vi "niDTS BT Rx Test INC Default Limits.vi"() -> ()   [LabVIEW 2015, in "niDTS BT.lvlib"]
uses:
  niDTS BT.lvlib
  niDTS BT Rx Test INC Results.ctl
panel:
  in  "Default BT RX LE USL":T1={"Total Packets Received (LE)"=2147483647, "Packets Sent (LE)"=inf, "Good Packets"=inf, "Packet Error Rate (%)"=30.8, "Error Bits"=4294967295, "Good Bits"=4294967295, "Total Received Bits"=4294967295, "Bit Error Rate (%)"=100.0}
  in  "Default BT RX LE LSL":T1
  in  "Default BT RX EDR USL":T1={"Total Packets Received (LE)"=2147483647, "Packets Sent (LE)"=inf, "Good Packets"=inf, "Packet Error Rate (%)"=100.0, "Error Bits"=4294967295, "Good Bits"=4294967295, "Total Received Bits"=4294967295, "Bit Error Rate (%)"=0.1}
  in  "Default BT RX EDR LSL":T1
  in  "Default BT RX BDR USL":T1={"Total Packets Received (LE)"=2147483647, "Packets Sent (LE)"=inf, "Good Packets"=inf, "Packet Error Rate (%)"=100.0, "Error Bits"=4294967295, "Good Bits"=4294967295, "Total Received Bits"=4294967295, "Bit Error Rate (%)"=0.007}
  in  "Default BT RX BDR LSL":T1
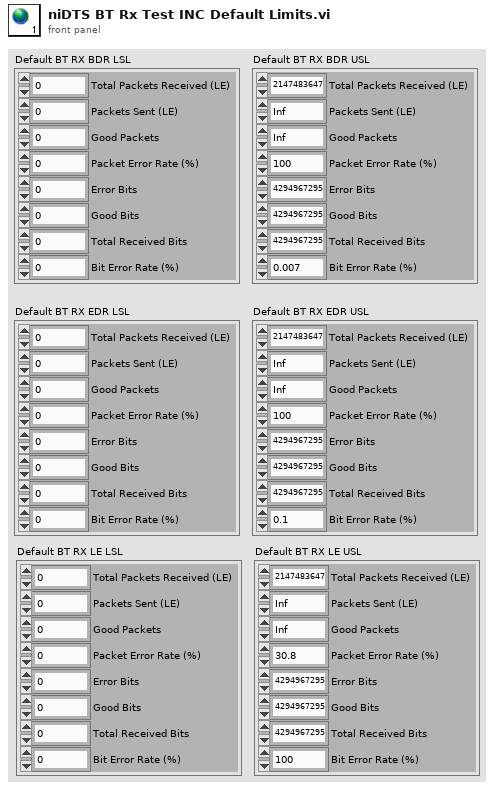
[diagram p1: front panel]
types:
  T1 = typedef "niDTS BT.lvlib/niDTS BT Rx Test INC Results.ctl" = cluster{"Total Packets Received (LE)":i32, "Packets Sent (LE)":dbl, "Good Packets":dbl, "Packet Error Rate (%)":dbl, "Error Bits":u32, "Good Bits":u32, "Total Received Bits":u32, "Bit Error Rate (%)":dbl}
diagram:
